vi "Untitled 2.vi"() -> ()   [LabVIEW 2024]
panel:
  in  "value":cluster{"String":string}
  out "Array 3":waveform(dbl)[](array[waveform])
  out "appended array":dbl[][](array[numeric])
  in  "Array 2":dbl[][](array[numeric])
  in  "Array":dbl[][](array[numeric])
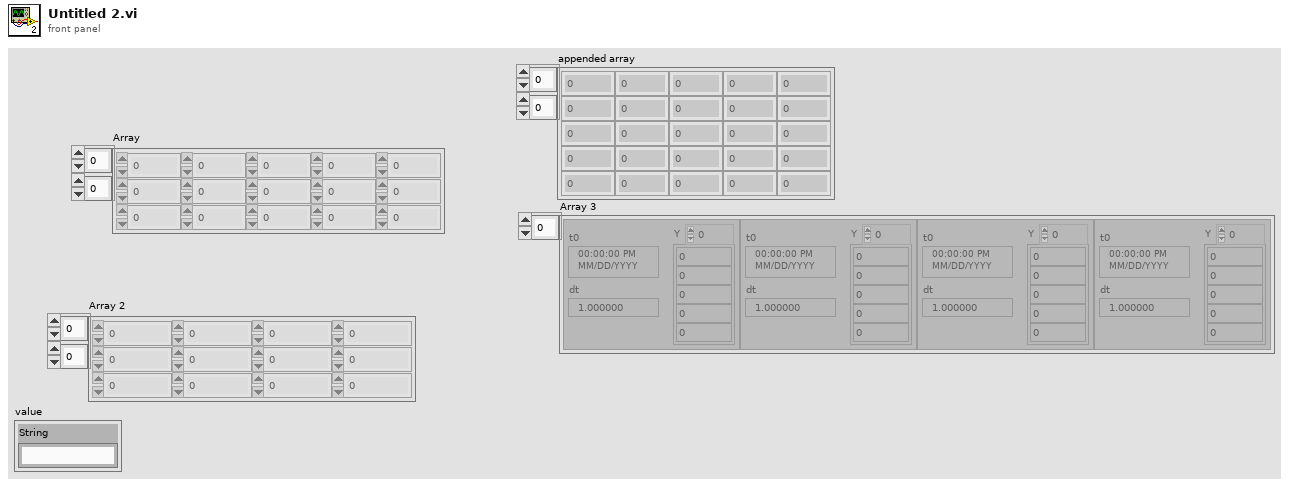
[diagram p1: front panel]
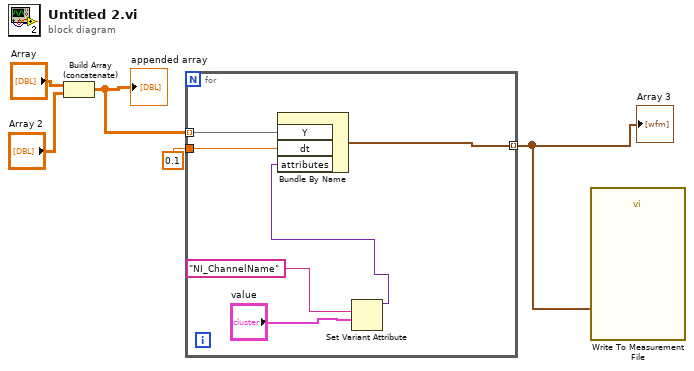
[diagram p0: block diagram]
diagram:
  n1 = Build Array (concatenate)("Array", "Array 2") -> (w3:dbl[][])
  "appended array" <- w3
  n2 = for {
    tunnel: w3 -> [w11] mode=indexing
    tunnel: 0.1 ("dt") -> [w10]
    tunnel: [w9] -> w1 mode=indexing
    n3 = Set Variant Attribute(name="NI_ChannelName", value="value") -> (Variant out=w8:variant)  [unwired: 2 in, 2 out]
    n4 = Bundle By Name("Y"=w11, "dt"=w10, "attributes"=w8) -> (w9:waveform(dbl))  [unwired: 1 in]
  }
  "Array 3" <- w1
  n5 = call "Write To Measurement File"("Signals"=w1) -> ()  [unwired: 16 in, 3 out]
